vi "Get frame rate.vi"(8 "error in (no error)":errorcluster, 11 "DAQOrcaFlash in":refnum<class "DAQOrcaFlash.lvclass">) -> (0 "error out":errorcluster, 3 "DAQOrcaFlash out":refnum<class "DAQOrcaFlash.lvclass">)   [LabVIEW 2012, in "DAQOrcaFlash.lvclass"]
uses:
  DAQOrcaFlash.lvclass
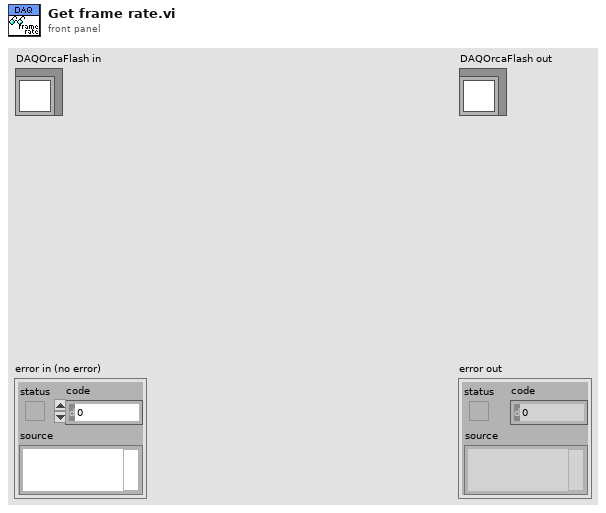
[diagram p1: front panel]
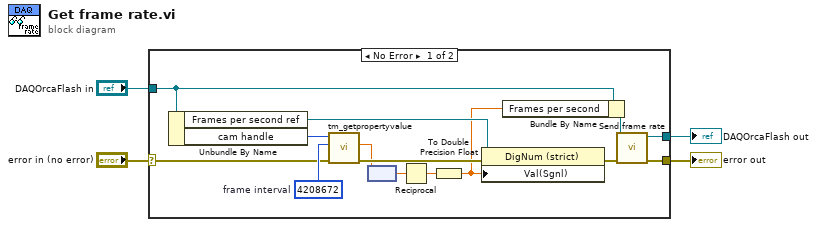
[diagram p0: block diagram]
diagram:
  n1 = case shown="No Error" "error in (no error)" {
    selector: "error in (no error)" -> [w11 w20]
    tunnel: [w15 w20] -> w3
    tunnel: [w13 w19] -> w1
    tunnel: "DAQOrcaFlash in" -> [w18 w19]
    frame No Error {
      w12 = u32 4208672  # frame interval
      n2 = Unbundle By Name(w18) -> ("Frames per second ref"=w17:refnum<vi>, "cam handle"=w10:u32)
      n3 = call <userlib>:"tm_getpropertyvalue.vi"("error in (no error)"=w11, "Property ID"=w12, "Handle in"=w10) -> ("error out"=w9:errorcluster, "Value in"=w8:sgl)  [unwired: 6 in, 1 out]
      n4 = node(w8) -> (w7:sgl[unit])
      n5 = Reciprocal(x=w7) -> (1/x=w6:sgl[unit])
      n6 = To Double Precision Float(number=w6) -> (double precision float=w5:dbl[unit])
      n7 = property class="DigNum (strict)"(reference=w17, error in=w9, "Val(Sgnl)"=w5) -> (error out=w16:errorcluster)  [unwired: 1 out]
      n8 = Bundle By Name(cluster=w18, "Frames per second"=w5) -> (w14:refnum<class "DAQOrcaFlash.lvclass">)
      n9 = call-dynamic "Send frame rate.vi"("error in (no error)"=w16, "DAQOrcaFlash in"=w14) -> ("error out"=w15:errorcluster, "DAQOrcaFlash out"=w13:refnum<class "DAQOrcaFlash.lvclass">)  [unwired: 8 in]
    }
    frame Error {
    }
  }
  "error out" <- w3
  "DAQOrcaFlash out" <- w1
